vi "Terminated.vi"(7 "Sender":refnum<class "Sender.lvclass">, 9 "Error":errorcluster, 10 "Actor":refnum<class "Actor.lvclass">, 11 "Terminated in":refnum<class "Terminated.lvclass">) -> (0 "Error out":errorcluster, 3 "Terminated out":refnum<class "Terminated.lvclass">)   [LabVIEW 2025, in "jettl.lvlib" / "Terminated Msg.lvlib" / "Terminated.lvclass"]
uses:
  Terminated.lvclass
  Actor/Actor/Actor.lvclass
  Sender/Sender/Sender.lvclass
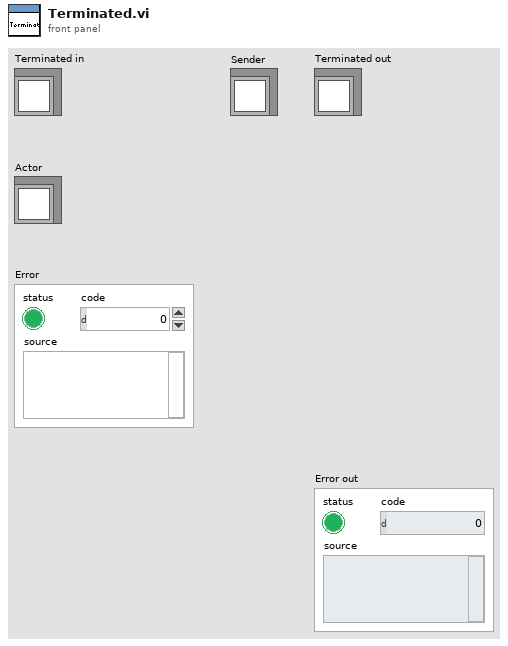
[diagram p1: front panel]
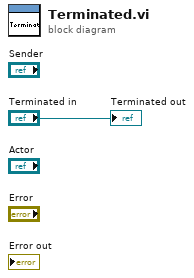
[diagram p0: block diagram]
diagram:
  "Terminated out" <- "Terminated in"
